vi "BIO_puts_low_level.vi"(8 "error in (no error)":errorcluster, 10 "Bytes to write":u8[](array[numeric]), 11 "BIO in":refnum<class "BIO.lvclass">) -> (0 "error out":errorcluster, 2 "return type":i32, 3 "BIO out":refnum<class "BIO.lvclass">)   [LabVIEW 2013, in "OpenSSL Socket.lvlib" / "BIO.lvclass"]
uses:
  BIO.lvclass
  SSL-Lib/SSL-Lib.lvclass/SSL-Lib.ctl
  BIO.lvclass/BIO.ctl
  SSL-Lib/Read Crypto Library Path.vi
  Read Handle.vi
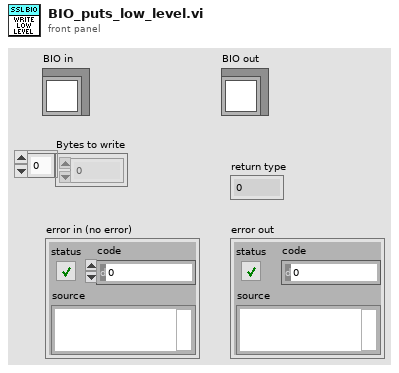
[diagram p1: front panel]
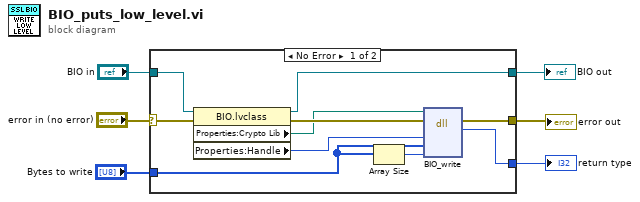
[diagram p0: block diagram]
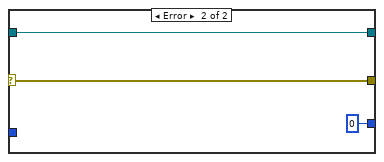
[diagram p2: hidden frame]
diagram:
  n1 = case shown="No Error" "error in (no error)" {
    selector: "error in (no error)" -> [w14 w18]
    tunnel: [w16 w18] -> w6
    tunnel: [w15 0 ("return type")] -> w5
    tunnel: "Bytes to write" -> [w8 _]
    tunnel: "BIO in" -> [w10 w19]
    tunnel: [w9 w19] -> w1
    frame No Error {
      n2 = property class="BIO.lvclass"(reference=w10, error in=w14) -> (reference out=w9:refnum<class "BIO.lvclass">, error out=w13:errorcluster, "Properties:Crypto Lib"=w12:path, "Properties:Handle"=w11:u64)
      n3 = Array Size(array=w8) -> (size(s)=w7:i32)
      n4 = dll-call lib="C:/Program Files (x86)/National Instruments/Shared/nissl/NIlibeay32.dll" fn="BIO_write"(path in=w12, error in=w13, "BIO"=w11, "buf"=w8, "len"=w7) -> (error out=w16:errorcluster, "return type"=w15:i32)  [unwired: 4 in, 1 out]
    }
    frame Error {
    }
  }
  "error out" <- w6
  "return type" <- w5
  "BIO out" <- w1
